vi "Get Supported Targets.vi"(8 "error in":errorcluster, 11 "configuration in":refnum<class "action configuration.lvclass">) -> (0 "error out":errorcluster, 2 "supported targets":T1[](array[typedef]), 3 "configuration out":refnum<class "action configuration.lvclass">)   [LabVIEW 2014, in "action configuration.lvclass"]
doc: "Provides an interface for determining the targets supported by a given configuration/runtime class pairing. This should be overridden by any useful child class."
uses:
  action configuration.lvclass
  <vilib>/NI/Tag Bus Module Framework/root configuration/Target Types.ctl
  <vilib>/NI/Tag Bus Module Framework/root configuration/TBM configuration.lvclass
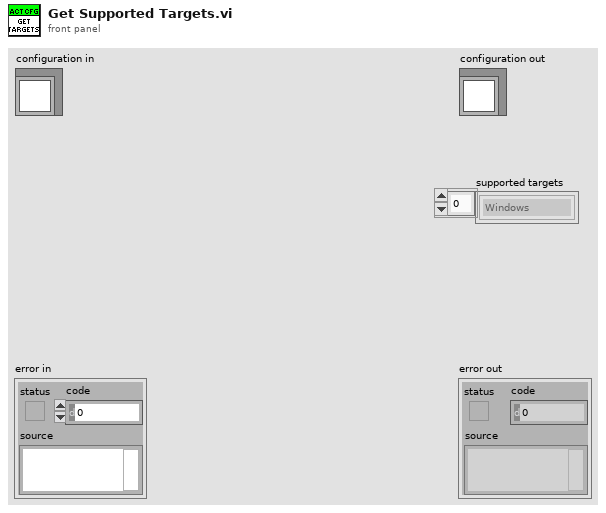
[diagram p1: front panel]
types:
  T1 = typedef "TBM configuration.lvclass/Target Types.ctl" = enum16{"Windows", "Mac", "Linux", "Linux RT ARM", "VxWorks", "Pharlap", "Other", "Linux RT x64"}
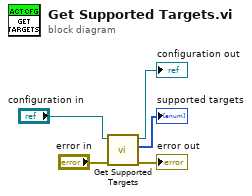
[diagram p0: block diagram]
diagram:
  n1 = call-parent "Get Supported Targets.vi"("error in"="error in", "configuration in"="configuration in") -> ("error out"=→"error out":errorcluster, "supported targets"=→"supported targets":T1[], "configuration out"=→"configuration out":refnum<class "action configuration.lvclass">)  [unwired: 7 in]
